vi "Read Oscilloscope.vi"(8 "error in (no error)":errorcluster caption="entrée d'erreur (pas d'erreur)", 11 "Control-Server en entrée":refnum<class "Control-Server.lvclass">) -> (0 "error out":errorcluster caption="sortie d'erreur", 2 "Oscilloscope.lvclass":refnum<class "Oscilloscope.lvclass">, 3 "Control-Server en sortie":refnum<class "Control-Server.lvclass">)   [LabVIEW 2015, in "Control-Server.lvclass"]
uses:
  Control-Server.lvclass
  Oscilloscope/Oscilloscope.lvclass
  Control-Server.lvclass/Control-Server.ctl
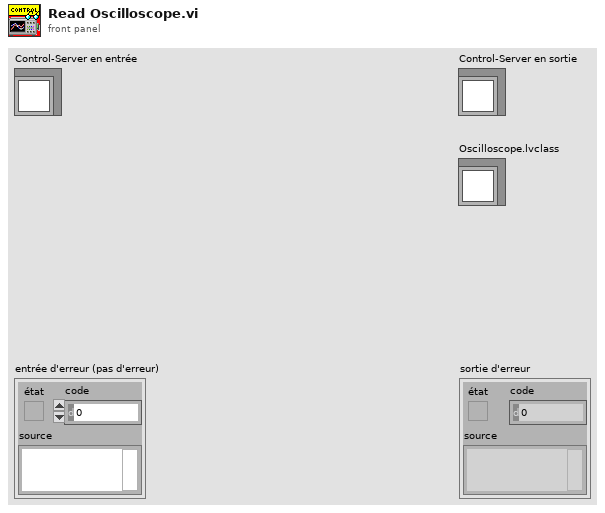
[diagram p1: front panel]
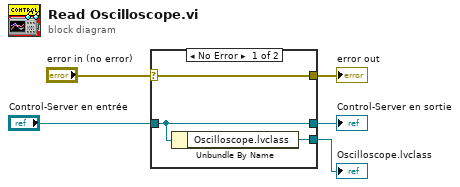
[diagram p0: block diagram]
diagram:
  n1 = case shown="No Error" "error in (no error)" {
    selector: "error in (no error)" -> [w8 w9]
    tunnel: [w8 w9] -> w4
    tunnel: [w7 w10] -> w2
    tunnel: "Control-Server en entrée" -> [w7 w10]
    tunnel: [w6 _] -> w1
    frame No Error {
      n2 = Unbundle By Name(w7) -> ("Oscilloscope.lvclass"=w6:refnum<class "Oscilloscope.lvclass">)
    }
    frame Error {
    }
  }
  "error out" <- w4
  "Control-Server en sortie" <- w2
  "Oscilloscope.lvclass" <- w1
